vi "FinalizingTurn.vi"(6 "Error":errorcluster, 10 "Message":refnum<class "Message.lvclass">, 11 "Actor":refnum<class "Actor.lvclass">) -> (2 "ProceedToTearingDown":bool, 3 "Actor":refnum<class "Actor.lvclass">, 4 "Error":errorcluster)   [LabVIEW 2020, in "jettl.lvlib"]
uses:
  jettl.lvlib
  Actor/Actor.lvclass
  Message/Message.lvclass
  Lifetime.ctl
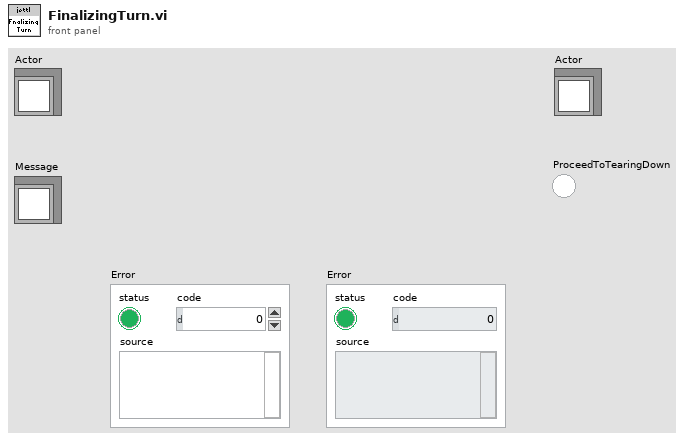
[diagram p1: front panel]
types:
  T1 = typedef "jettl.lvlib/Lifetime.ctl" = enum16{"Init", "Spawn", "Setup", "TeardownBeforeRunning", "Running", "StopCalled", "StoppingWithComponents", "StoppingNoComponents", "TeardownAfterRunning", "Stopped"}
  T2 = typedef "jettl.lvlib/BaseActor.ctl" = cluster{"Lifetime":T1, "SelfActor":T3, "MediatorActor":T3, "ComponentActorMap":T8}
  T3 = typedef "jettl.lvlib/Actor.ctl" = cluster{"Messages":T4, "ActorAlias":string, "ActorType":T7, "Transport":refnum<user-event>, "Address":refnum<event-registration>, "VIRef":refnum<vi>}
  T4 = typedef "jettl.lvlib/Messages.ctl" = cluster{"Listen":T5, "TellSelf":T5, "TellMediator":T5, "TellComponentMap":T6}
  T5 = typedef "jettl.lvlib/MessageSet.ctl" = set{refnum<class "Message.lvclass">}
  T6 = typedef "jettl.lvlib/TellComponentMap.ctl" = map{string, T5}
  T7 = typedef "jettl.lvlib/ActorType.ctl" = enum16{"Mediator", "Component"}
  T8 = typedef "jettl.lvlib/ComponentActorMap.ctl" = map{string, T3}
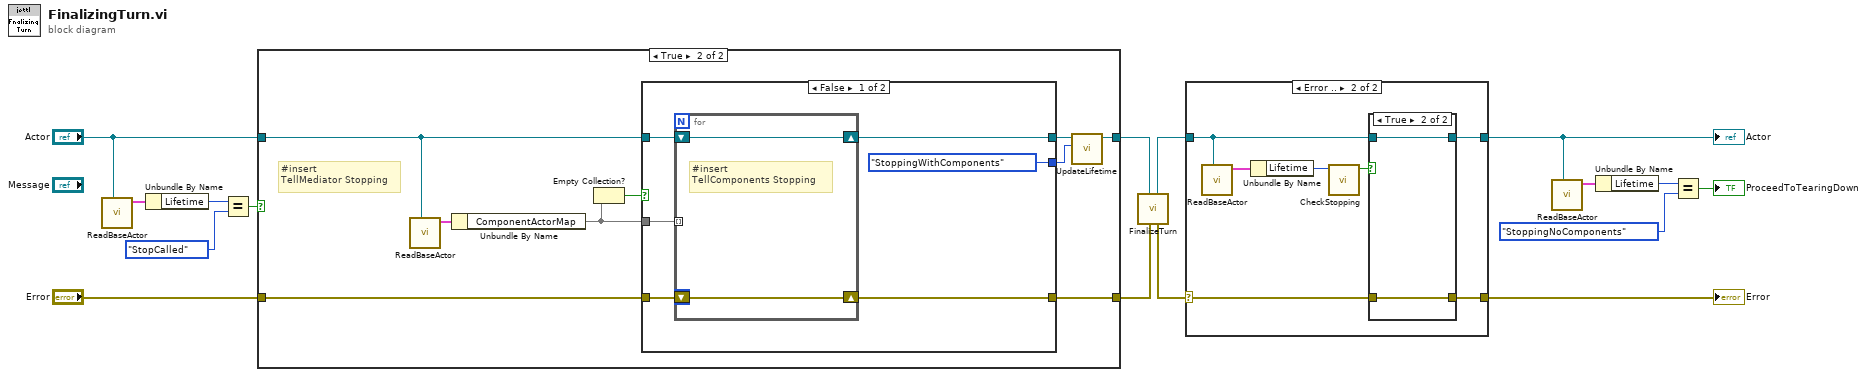
[diagram p0: block diagram]
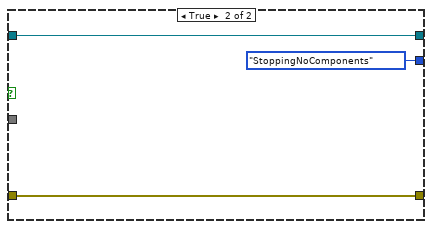
[diagram p3: hidden frame]
diagram:
  n1 = call-dynamic "ReadBaseActor.vi"("Actor"="Actor") -> ("BaseActor"=w13:T2)  [unwired: 10 in]
  n2 = Unbundle By Name(w13) -> ("Lifetime"=w12:T1)
  n3 = Equal?(x=w12, y=Lifetime."StopCalled") -> (x = y?=w15:bool)
  n4 = case shown="True" w15 {
    tunnel: "Error" -> [w18 w25]
    tunnel: [w18 w27] -> w4
    tunnel: [w17 w24] -> w5
    tunnel: "Actor" -> [w17 w21]
    frame False {
    }
    frame True {
      # "#insert\nTellMediator Stopping"
      n5 = call-dynamic "ReadBaseActor.vi"("Actor"=w21) -> ("BaseActor"=w20:T2)  [unwired: 10 in]
      n6 = Unbundle By Name(w20) -> ("ComponentActorMap"=w19:T8)
      n7 = Empty Collection?(1:w19) -> (0:w26:bool)
      n8 = case shown="False" w26 {
        tunnel: w25 -> [w33 w37]
        tunnel: [w32 w37] -> w27
        tunnel: [Lifetime."StoppingWithComponents" ("Lifetime") Lifetime."StoppingNoComponents" ("Lifetime")] -> w22
        tunnel: w21 -> [w31 w38]
        tunnel: [w30 w38] -> w23
        tunnel: w19 -> [w29 _]
        frame False {
          n9 = for {
            tunnel: w29 -> [_] mode=indexing
            shift-right: [w34] -> w32
            shift-left: w33 -> [w34]
            shift-right: [w35] -> w30
            shift-left: w31 -> [w35]
            # "#insert\nTellComponents Stopping"
          }
        }
        frame True {
        }
      }
      n10 = call "UpdateLifetime.vi"("Lifetime"=w22, "Actor"=w23) -> ("Actor"=w24:refnum<class "Actor.lvclass">)  [unwired: 9 in]
    }
  }
  n11 = call-dynamic "FinalizeTurn.vi"("Error"=w4, "Actor"=w5) -> ("Error"=w3:errorcluster, "Actor"=w2:refnum<class "Actor.lvclass">)  [unwired: 8 in]
  n12 = case shown="Error .." w3 {
    selector: w3 -> [_ w45]
    tunnel: [_ w46] -> w16
    tunnel: w2 -> [w39 w42]
    tunnel: [w39 w40] -> w1
    frame No Error {
    }
    frame Error {
      n13 = call-dynamic "ReadBaseActor.vi"("Actor"=w42) -> ("BaseActor"=w44:T2)  [unwired: 10 in]
      n14 = Unbundle By Name(w44) -> ("Lifetime"=w43:T1)
      n15 = call "CheckStopping.vi"("Lifetime"=w43) -> ("Stopping"=w41:bool)  [unwired: 10 in]
      n16 = case shown="True" w41 {
        tunnel: [w48 w50] -> w40
        tunnel: w42 -> [w48 w50]
        tunnel: w45 -> [w47 w49]
        tunnel: [w47 w49] -> w46
        frame False {
          # "#insert\nTellSelf Stop"
        }
        frame True {
        }
      }
    }
  }
  "Actor" <- w1
  "Error" <- w16
  n17 = call-dynamic "ReadBaseActor.vi"("Actor"=w1) -> ("BaseActor"=w9:T2)  [unwired: 10 in]
  n18 = Unbundle By Name(w9) -> ("Lifetime"=w8:T1)
  n19 = Equal?(x=w8, y=Lifetime."StoppingNoComponents") -> (x = y?=→"ProceedToTearingDown":bool)
